vi "I2C_WriteByte Example.vi"(3 "error in":errorcluster, 4 "Address":u8 format="%.0x", 5 "Bus":i32=1, 6 "Byte":u8 format="%.0x") -> (10 "error out":errorcluster)   [LabVIEW 2014]
doc: "This example VI demonstrates writing a single byte to a device connected to the I2C bus."
uses:
  GPIO.lvlib
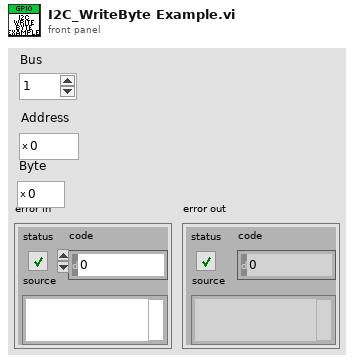
[diagram p1: front panel]
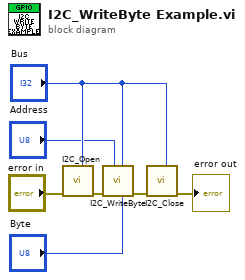
[diagram p0: block diagram]
diagram:
  n1 = call "I2C_Open.vi"("Bus"="Bus", "error in"="error in") -> ("error out"=w5:errorcluster)  [unwired: 9 in]
  n2 = call "I2C_WriteByte.vi"("Byte"="Byte", "Bus"="Bus", "Address"="Address", "error in"=w5) -> ("error out"=w3:errorcluster)  [unwired: 7 in]
  n3 = call "I2C_Close.vi"("Bus"="Bus", "error in"=w3) -> ("error out"=→"error out":errorcluster)  [unwired: 9 in]
